vi "test_ExistingClientConnection_StopPinMapService_UpdatePinMapFromXMLWorksWithoutError.vi"(8 "error in":errorcluster) -> (0 "error out":errorcluster, 2 "result":string, 3 "pass":bool)   [LabVIEW 2021, in "MeasurementServerTests.lvlib" / "Pin Map Tests.lvlib"]
uses:
  Pin Map Tests.lvlib
  gRPC/Generated APIs/ni/measurementlink/pinmap/v1/RPC Messages/ni_measurementlink_pinmap_v1_UpdatePinMapFromXmlRequest.ctl
  Helpers/Pin Map XML Strings Global.vi
  MeasurementServerTests.lvlib
  Runtime/Clients/Pin Map V1/NI Pin Map V1 Client.lvlib
  gRPC/Generated APIs/ni/measurementlink/pinmap/v1/ni.measurementlink.pinmap.v1.api.lvlib
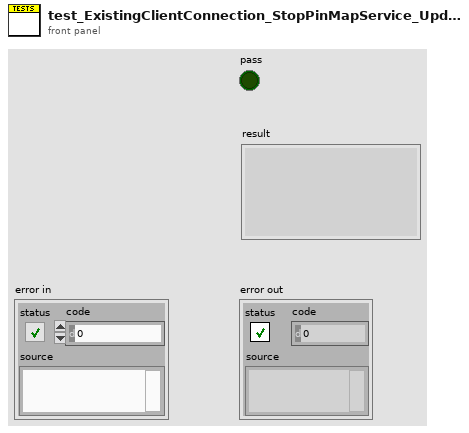
[diagram p1: front panel]
types:
  T1 = typedef "ni.measurementlink.pinmap.v1.api.lvlib/ni_measurementlink_pinmap_v1_UpdatePinMapFromXmlRequest.ctl" = cluster{"pin_map_id":string, "pin_map_xml":string}
  T2 = typedef "ni.measurementlink.pinmap.v1.api.lvlib/ni_measurementlink_pinmap_v1_PinMap.ctl" = cluster{"pin_map_id":string}
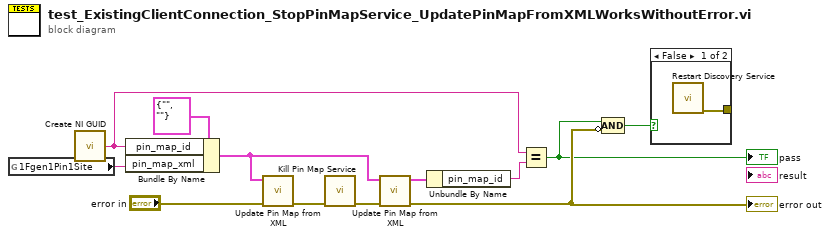
[diagram p0: block diagram]
diagram:
  n1 = global read "Pin Map XML Strings Global.vi" "1Fgen1Pin1Site"() -> (w3:string)
  n2 = call <vilib>:"Create NI GUID.vi"() -> ("NI GUID"=w1:string)
  n3 = Bundle By Name(cluster=T1 {"pin_map_id"="", "pin_map_xml"=""} ("Request Data"), "pin_map_id"=w1, "pin_map_xml"=w3) -> (w2:T1)
  n4 = call "Update Pin Map from XML.vi"("error in"="error in", "request data"=w2) -> ("error out"=w5:errorcluster)  [unwired: 8 in, 1 out]
  n5 = call "Kill Pin Map Service.vi"("error in"=w5) -> ("error out"=w10:errorcluster)  [unwired: 10 in]
  n6 = call "Update Pin Map from XML.vi"("error in"=w10, "request data"=w2) -> ("error out"=w11:errorcluster, "response data"=w9:T2)  [unwired: 8 in]
  "error out" <- w11
  n7 = Unbundle By Name(w9) -> ("pin_map_id"=w8:string)
  n8 = Equal?(x=w1, y=w8) -> (x = y?=w7:bool)
  "pass" <- w7
  n9 = Compound Arithmetic op=AND(w7, invert w11) -> (w12:bool)
  n10 = case shown="False" w12 {
    tunnel: [w13 _] -> _
    frame False {
      n11 = call "Restart Discovery Service.vi"() -> ("error out"=w13:errorcluster)  [unwired: 11 in]
    }
    frame True {
    }
  }
